vi "XMLparser.vi"(1 "XML File Path":path, 2 "Array":string[](array[string])) -> (0 "toArrayParser":string[][](array[string]))   [LabVIEW 2010]
uses:
  <vilib>/xml/NI_XML.lvlib
  E:/Program Files (x86)/National Instruments/LabVIEW 2010/resource/objmgr/DOMUserDefRef.rc
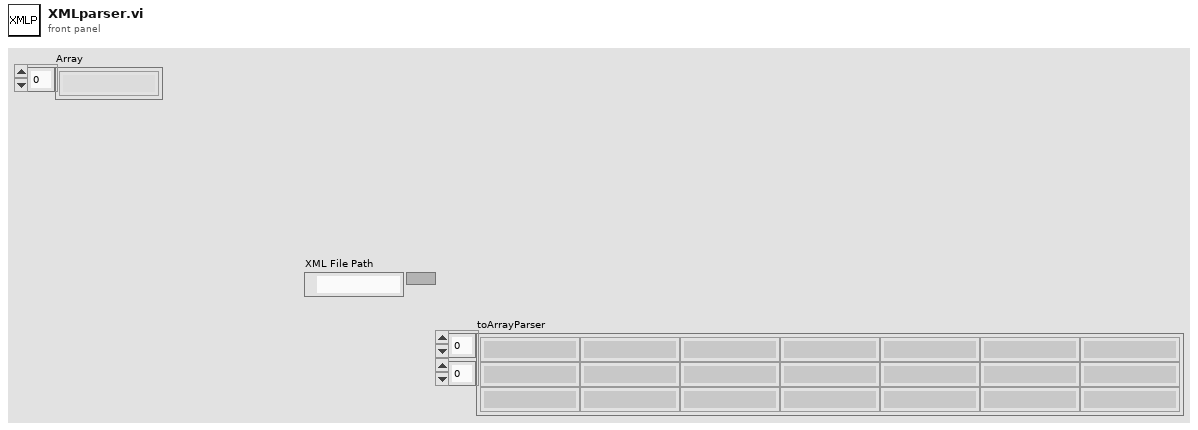
[diagram p1: front panel]
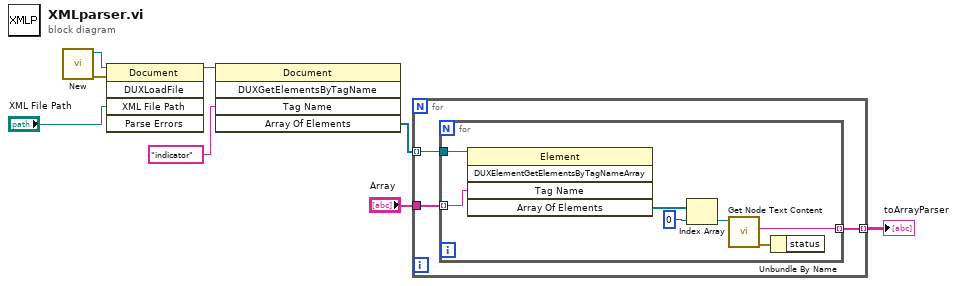
[diagram p0: block diagram]
diagram:
  n1 = call <vilib>:"New.vi"() -> ("error out"=w7:errorcluster, "DOM document out"=w8:refnum<k20>)  [unwired: 8 in]
  n2 = invoke class="Document" method="DUXLoadFile"(reference=w8, error in=w7, "XML File Path"="XML File Path") -> (reference out=w5:refnum<k20>)  [unwired: 2 in, 4 out]
  n3 = invoke class="Document" method="DUXGetElementsByTagName"(reference=w5, "Tag Name"="indicator") -> ("Array Of Elements"=w4:refnum<k20>[])  [unwired: 3 in, 4 out]
  n4 = for {
    tunnel: "Array" -> [w9]
    tunnel: [w11] -> w3 mode=indexing
    tunnel: w4 -> [w10] mode=indexing
    n5 = for {
      tunnel: [w18] -> w11 mode=indexing
      tunnel: w10 -> [w17]
      tunnel: w9 -> [w13] mode=indexing
      n6 = invoke class="Element" method="DUXElementGetElementsByTagNameArray"(reference=w17, "Tag Name"=w13) -> ("Array Of Elements"=w15:refnum<k20>[])  [unwired: 3 in, 4 out]
      n7 = Index Array(array=w15, index=0) -> (element=w16:refnum<k20>)
      n8 = call <vilib>:"Get Node Text Content.vi"("node in"=w16) -> ("error out"=w12:errorcluster, "node text"=w18:string)  [unwired: 8 in, 1 out]
      n9 = Unbundle By Name(w12) -> ()  [unwired: 1 out]
    }
  }
  "toArrayParser" <- w3
